vi "BK Precision 8600 Series Run Constant Resistance Transient.vi"() -> ()   [LabVIEW 2018]
doc: "Exemplifies how to configure and run a constant resistance transient operation in which the load will continuously toggle between level A and level B value with the specified time."
uses:
  <instrlib>/BK Precision 8600 Series/BK Precision 8600 Series.lvlib
panel:
  in  "B Level Value (2)":dbl=2.0 min=0.0 max=7500.0 step=1.0 format="%.3f"
  in  "A Level Value (1)":dbl=1.0 min=0.0 max=7500.0 step=1.0 format="%.3f"
  in  "?":bool
  in  "A Width (1)":dbl=1.0 min=0.0 max=120.0 step=1.0 format="%#.3f"
  in  "B Width (1)":dbl=1.0 min=0.0 max=120.0 step=1.0 format="%#.3f"
  in  "VISA resource name":refnum<visa-resource-name>
  in  "Serial Configuration":cluster{"Baud Rate":u32}={"Baud Rate"=9600} {"Baud Rate" items=["300"=300, "600"=600, "1200"=1200, "2400"=2400, "4800"=4800, "9600"=9600, "19200"=19200]}
  # "(c) 2014-2019 B&K Precision Corporation.  ALL RIGHTS RESERVED."
  # "ohm"
  # "ohm"
  # "s"
  # "s"
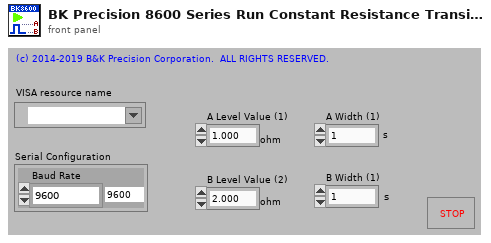
[diagram p1: front panel]
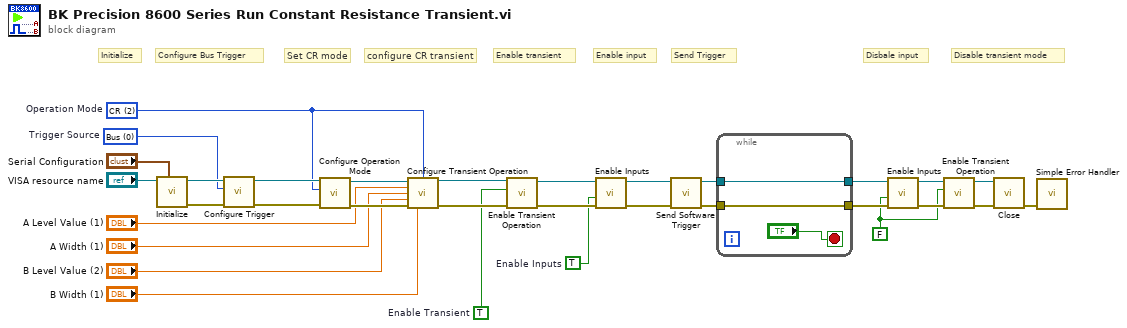
[diagram p0: block diagram]
diagram:
  w3 = u16 2 items=["CC", "CV", "CR", "CW", "CZ"]  # Operation Mode
  w4 = u16 0 items=["Bus", "External", "Hold", "Manual", "Timed"]  # Trigger Source
  w5 = FALSE
  w12 = TRUE  # Enable Inputs
  w20 = TRUE  # Enable Transient
  # "Disable transient mode"
  # "Disbale input"
  # "Send Trigger"
  # "Enable input"
  # "Enable transient"
  # "configure CR transient"
  # "Set CR mode"
  # "Configure Bus Trigger"
  # "Initialize"
  n1 = call <instrlib>:"Initialize.vi"("Serial Configuration"="Serial Configuration", "VISA resource name"="VISA resource name") -> ("error out"=w29:errorcluster, "VISA resource name out"=w30:refnum<visa-resource-name>)  [unwired: 8 in]
  n2 = call <instrlib>:"Configure Trigger.vi"("error in (no error)"=w29, "Trigger Source (0:Bus)"=w4, "VISA resource name"=w30) -> ("error out"=w27:errorcluster, "VISA resource name out"=w28:refnum<visa-resource-name>)  [unwired: 7 in]
  n3 = call <instrlib>:"Configure Operation Mode.vi"("error in (no error)"=w27, "Operation Mode (0:CC)"=w3, "VISA resource name"=w28) -> ("error out"=w25:errorcluster, "VISA resource name out"=w26:refnum<visa-resource-name>)  [unwired: 7 in]
  n4 = call <instrlib>:"Configure Transient Operation.vi"("VISA resource name"=w26, "Transient Type (0:CC)"=w3, "A Level Value (1)"="A Level Value (1)", "A Width (1)"="A Width (1)", "B Level Value (2)"="B Level Value (2)", "error in (no error)"=w25, "B Width (1)"="B Width (1)") -> ("VISA resource name out"=w22:refnum<visa-resource-name>, "error out"=w21:errorcluster)  [unwired: 7 in]
  n5 = call <instrlib>:"Enable Transient Operation.vi"("error in (no error)"=w21, "Enable Transient (T: Enable)"=w20, "VISA resource name"=w22) -> ("error out"=w16:errorcluster, "VISA resource name out"=w15:refnum<visa-resource-name>)  [unwired: 7 in]
  n6 = call <instrlib>:"Enable Inputs.vi"("error in (no error)"=w16, "Enable Input (F: False)"=w12, "VISA resource name"=w15) -> ("error out"=w13:errorcluster, "VISA resource name out"=w14:refnum<visa-resource-name>)  [unwired: 7 in]
  n7 = call <instrlib>:"Send Software Trigger.vi"("error in (no error)"=w13, "VISA resource name"=w14) -> ("error out"=w18:errorcluster, "VISA resource name out"=w19:refnum<visa-resource-name>)  [unwired: 8 in]
  n8 = while {
    tunnel: [w34] -> w11
    tunnel: w19 -> [w34]
    tunnel: [w33] -> w10
    tunnel: w18 -> [w33]
    stop <- "?" stop-if-true
  }
  n9 = call <instrlib>:"Enable Inputs.vi"("error in (no error)"=w10, "Enable Input (F: False)"=w5, "VISA resource name"=w11) -> ("error out"=w9:errorcluster, "VISA resource name out"=w8:refnum<visa-resource-name>)  [unwired: 7 in]
  n10 = call <instrlib>:"Enable Transient Operation.vi"("error in (no error)"=w9, "Enable Transient (T: Enable)"=w5, "VISA resource name"=w8) -> ("error out"=w6:errorcluster, "VISA resource name out"=w7:refnum<visa-resource-name>)  [unwired: 7 in]
  n11 = call <instrlib>:"Close.vi"("error in (no error)"=w6, "VISA resource name"=w7) -> ("error out"=w17:errorcluster)  [unwired: 9 in]
  n12 = call <vilib>:"Simple Error Handler.vi"("error in (no error)"=w17) -> ()  [unwired: 4 in, 5 out]
